vi "HashTable Demo1.vi"() -> ()   [LabVIEW 2011]
uses:
  HashTable.lvclass
panel:
  out "Values":variant[](array[variant])
  out "Keys":variant[](array[variant])
  out "New Count":i32
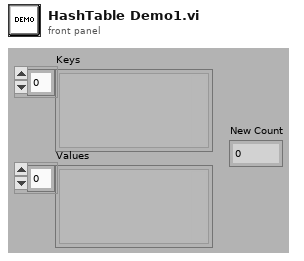
[diagram p1: front panel]
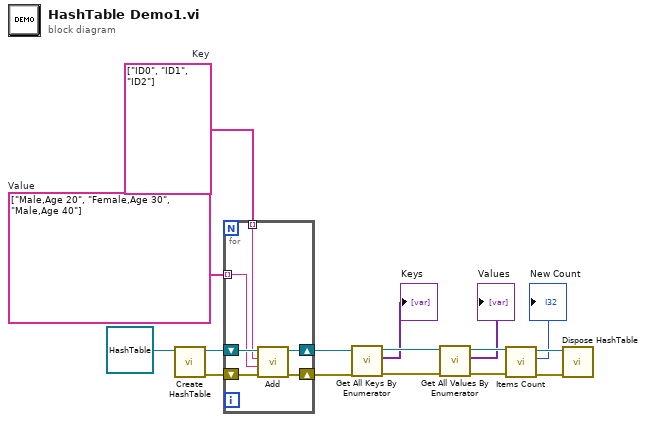
[diagram p0: block diagram]
diagram:
  w13 = string[] ["Male,Age 20", "Female,Age 30", "Male,Age 40"]  # Value
  w12 = string[] ["ID0", "ID1", "ID2"]  # Key
  n1 = call "Create HashTable.vi"("HashTable 输入"=refnum<class "HashTable.lvclass"> refnum ("HashTable.lvclass")) -> ("error out"=w14:errorcluster, "HashTable 输出"=w15:refnum<class "HashTable.lvclass">)  [unwired: 9 in]
  n2 = for {
    tunnel: w12 -> [w18] mode=indexing
    shift-right: [w19] -> w8
    shift-left: w15 -> [w20]
    shift-right: [w21] -> w7
    shift-left: w14 -> [w22]
    tunnel: w13 -> [w17] mode=indexing
    n3 = call "Add.vi"("error in (no error)"=w22, "Value"=w17, "Key"=w18, "HashTable 输入"=w20) -> ("error out"=w21:errorcluster, "HashTable 输出"=w19:refnum<class "HashTable.lvclass">)  [unwired: 6 in]
  }
  n4 = call "Get All Keys By Enumerator.vi"("error in (no error)"=w7, "HashTable 输入"=w8) -> ("error out"=w5:errorcluster, "Keys"=→"Keys":variant[], "HashTable 输出"=w6:refnum<class "HashTable.lvclass">)  [unwired: 7 in]
  n5 = call "Get All Values By Enumerator.vi"("error in (no error)"=w5, "HashTable 输入"=w6) -> ("error out"=w3:errorcluster, "Values"=→"Values":variant[], "HashTable 输出"=w4:refnum<class "HashTable.lvclass">)  [unwired: 7 in]
  n6 = call "Items Count.vi"("error in (no error)"=w3, "HashTable 输入"=w4) -> ("error out"=w10:errorcluster, "Count"=→"New Count":i32, "HashTable 输出"=w11:refnum<class "HashTable.lvclass">)  [unwired: 7 in]
  n7 = call "Dispose HashTable.vi"("error in (no error)"=w10, "HashTable 输入"=w11) -> ()  [unwired: 8 in, 2 out]
